vi "U64toRgba_2D.vi"(11 "U64":u64[][](array[numeric])) -> (3 "Rgba":T1[][](array[typedef]))   [LabVIEW 2024, in "OpenLvVision_Image.lvlib" / "DataAccess.lvlib"]
doc: "Convert an number into an cluster"
uses:
  DataAccess.lvlib
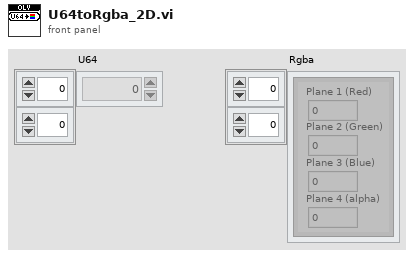
[diagram p1: front panel]
types:
  T1 = typedef "Color (U64)" = cluster{"Plane 3 (Blue)":u16, "Plane 2 (Green)":u16, "Plane 1 (Red)":u16, "Plane 4 (alpha)":u16}
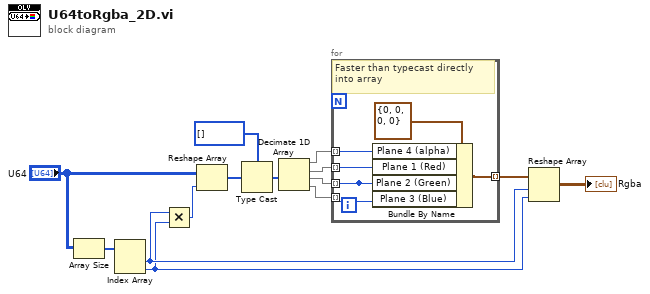
[diagram p0: block diagram]
diagram:
  n1 = Array Size(array="U64") -> (size(s)=w8:i32[])
  n2 = Index Array(array=w8) -> (element #1=w4:i32, element #2=w2:i32)  [unwired: 2 in]
  n3 = Multiply(x=w4, y=w2) -> (x*y=w3:i32)
  n4 = Reshape Array("U64", w3) -> (w5:u64[])
  n5 = Type Cast(type=u16[] [], x=w5) -> (*(type *) &x=w13:u16[])
  n6 = Decimate 1D Array(w13) -> (w12:u16[], w10:u16[], w9:u16[], w11:u16[])
  n7 = for {
    tunnel: w12 -> [w20] mode=indexing
    tunnel: w10 -> [w19] mode=indexing
    tunnel: [w16] -> _ mode=indexing
    tunnel: w11 -> [w18] mode=indexing
    tunnel: [w17] -> w7 mode=indexing
    tunnel: w9 -> [w16] mode=indexing
    # "Faster than typecast directly into array"
    n8 = Bundle By Name(cluster=T1 {"Plane 3 (Blue)"=0, "Plane 2 (Green)"=0, "Plane 1 (Red)"=0, "Plane 4 (alpha)"=0} ("Color"), "Plane 4 (alpha)"=w20, "Plane 1 (Red)"=w19, "Plane 2 (Green)"=w16, "Plane 3 (Blue)"=w18) -> (w17:T1)
  }
  n9 = Reshape Array(w7, w4, w2) -> (→"Rgba":T1[][])
